vi "PhotonCamera_SetLEDMode.vi"(9 "LEDMode":T1, 11 "BaseNTName":string="/photonvision") -> (0 "error out":errorcluster)   [LabVIEW 2019, in "PhotonVisionLib.lvlib"]
doc: "Sets the LED mode.\n\nInputs:\n - BaseNTName - string - Base Nework Table name. (Optional. Default: /photonvision )\n - LedMod -- The mode to set to.\n\nOutputs:\n - Error Out -- Contains error information if a Network table ot other error occured."
uses:
  PhotonVisionLib.lvlib
  Enum/VisionLEDModeType.ctl
  <vilib>/Rock Robotics/WPI/ThirdParty/JAS_Junk/TrajLib/VI/Util_GetTime_U32.vi
  <vilib>/Rock Robotics/WPI/ThirdParty/JAS_Junk/TrajLib/VI/Util_GetTime_U64.vi
  <vilib>/Rock Robotics/Network Tables/NT Read Integer.vi
  <vilib>/Rock Robotics/Network Tables/NT Read Boolean.vi
  <vilib>/Rock Robotics/Network Tables/NT Write Integer.vi
  <vilib>/Rock Robotics/WPI/ThirdParty/JAS_Junk/TrajLib/Trajectory_Library.lvlib
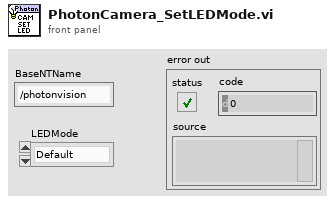
[diagram p1: front panel]
types:
  T1 = typedef "PhotonVisionLib.lvlib/VisionLEDModeType.ctl" = enum16{"Default", "Off", "On", "Blink"}
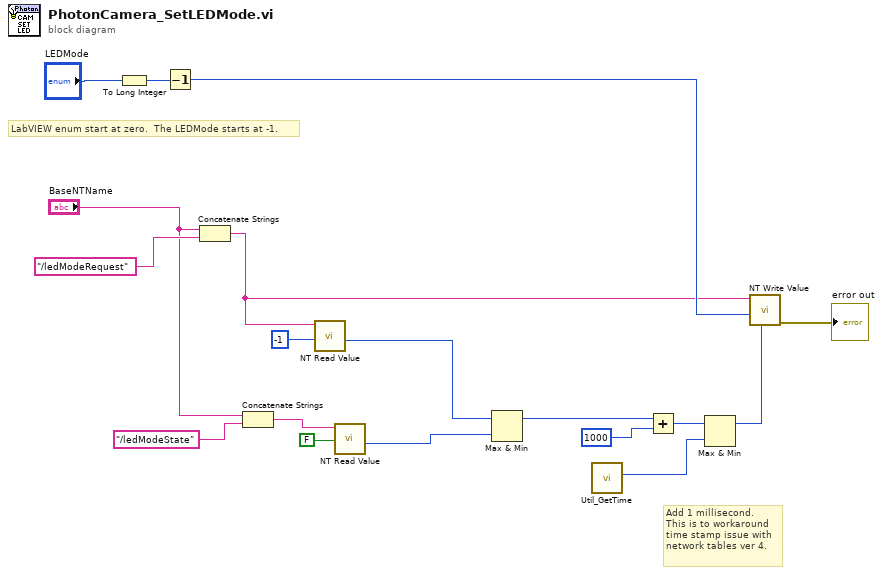
[diagram p0: block diagram]
diagram:
  # "Add 1 millisecond.\nThis is to workaround\ntime stamp issue with\nnetwork tables ver 4."
  # "LabVIEW enum start at zero.  The LEDMode starts at -1."
  n1 = To Long Integer(number="LEDMode") -> (32bit integer=w17:i32)
  n2 = Decrement(x=w17) -> (x-1=w11:i32)
  n3 = Concatenate Strings("BaseNTName", "/ledModeRequest") -> (w8:string)
  n4 = Concatenate Strings("BaseNTName", "/ledModeState") -> (w7:string)
  n5 = call-poly <vilib>:"NT Read Value.vi"("default value"=i64 -1 ("Default Value"), "name"=w8) -> ("timestamp"=w2:u64)  [unwired: 7 in, 2 out]
  n6 = call-poly <vilib>:"NT Read Value.vi"("default value"=FALSE ("Default Value"), "name"=w7) -> ("timestamp"=w5:u64)  [unwired: 7 in, 2 out]
  n7 = Max & Min(x=w2, y=w5) -> (max(x,y)=w1:u64)  [unwired: 1 out]
  n8 = call <vilib>:"Util_GetTime.vi"() -> ("FPGA_Time_MicroSeconds"=w14:u64)  [unwired: 9 in, 2 out]
  n9 = Add(x=w1, y=u64 1000) -> (x+y=w15:u64)
  n10 = Max & Min(x=w15, y=w14) -> (max(x,y)=w12:u64)  [unwired: 1 out]
  n11 = call-poly <vilib>:"NT Write Value.vi"("timestamp"=w12, "value"=w11, "name"=w8) -> ("error out"=→"error out":errorcluster)  [unwired: 8 in]
